vi "Tree.vi"   [LabVIEW 2011, in "Messenging.lvlib"]
doc: "Commonly used VI's."
uses:
  Messenging.lvlib
  Interprocess Messenger/QueueMessenger/QueueMessenger.lvclass
  Interprocess Messenger/EventMessenger/EventMessenger.lvclass
  Interprocess Messenger/Messenger (Parent)/MGR.lvclass
  Interprocess Messenger/Send/Send.lvclass
  Interprocess Messenger/Send/Send Message.vi
  Interprocess Messenger/TextVarientMessage/MSG.lvclass
  Parallel Process/Parallel Process.lvclass
  Parallel Process/Messsage Logger/Message Logger.lvclass
  Parallel Process/State Logger Folder/State Logger.lvclass
  Parallel Process/PP Template (Receive type)/PP Template.lvclass
  Parallel Process/PP Template (EventUI)/Parallel Process Template (EventUI) Folder/PP Template (UserEvent).lvclass
  Interprocess Messenger/SendMultiple/Create Observer.vi
  Interprocess Messenger/SendMultiple/ObserverSet.lvclass
  Interprocess Messenger/SendOnly/Observer.lvclass
  Parallel Process/ObserverRegister/ObserverRegistry.lvclass
  Parallel Process/ObserverRegister/Menu/Notify Observers (State).vi
  Interprocess Messenger/Cancelable Observer/CancelableObserver.lvclass
  Parallel Process/Metronome/Metronome.lvclass
  Interprocess Messenger/TextVarientMessage/Reply (message).vi
  Interprocess Messenger/TextVarientMessage/Write (no data).vi
  Interprocess Messenger/Send/Query (static).vi
  Parallel Process/Attach Observer.vi
  Interprocess Messenger/Receiver/MGR (Receive type).lvclass
  Interprocess Messenger/VarMessage/Extract Varient (static).vi
panel:
  # "See diagram"
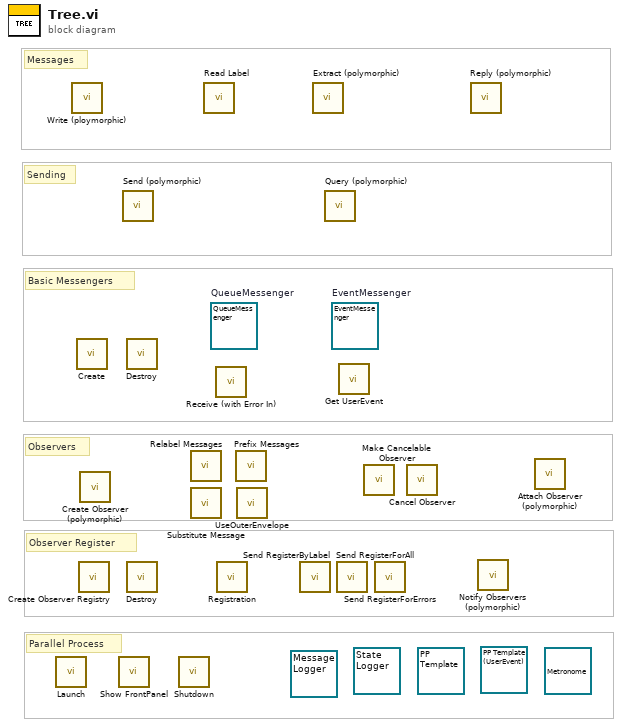
[diagram p0: block diagram]
diagram:
  (unwired) refnum<class "Metronome.lvclass"> refnum ("Messenging.lvlib:Metronome.lvclass")
  (unwired) refnum<class "PP Template (UserEvent).lvclass"> refnum ("Messenging.lvlib:PP Template (UserEvent).lvclass")
  (unwired) refnum<class "PP Template.lvclass"> refnum ("Messenging.lvlib:PP Template.lvclass")
  (unwired) refnum<class "State Logger.lvclass"> refnum ("Messenging.lvlib:State Logger.lvclass")
  (unwired) refnum<class "Message Logger.lvclass"> refnum ("Messenging.lvlib:Message Logger.lvclass")
  (unwired) refnum<class "EventMessenger.lvclass"> refnum  # EventMessenger
  (unwired) refnum<class "QueueMessenger.lvclass"> refnum  # QueueMessenger
  # "Parallel Process"
  # "Observer Register"
  # "Observers"
  # "Basic Messengers"
  # "Sending"
  # "Messages"
  n1 = call-dynamic "Launch.vi"() -> ()  [unwired: 9 in, 3 out]
  n2 = call-poly "Write (ploymorphic).vi"() -> ()  [unwired: 10 in, 2 out]
  n3 = call-dynamic "Create.vi"() -> ()  [unwired: 10 in, 2 out]
  n4 = call "Create Observer Registry.vi"() -> ()  [unwired: 10 in, 2 out]
  n5 = call-poly "Create Observer (polymorphic).vi"() -> ()  [unwired: 9 in, 1 out]
  n6 = call-dynamic "Show FrontPanel.vi"() -> ()  [unwired: 10 in, 2 out]
  n7 = call-poly "Send (polymorphic).vi"() -> ()  [unwired: 10 in, 2 out]
  n8 = call-dynamic "Destroy.vi"() -> ()  [unwired: 11 in, 1 out]
  n9 = call "Destroy.vi"() -> ()  [unwired: 10 in, 2 out]
  n10 = call-dynamic "Shutdown.vi"() -> ()  [unwired: 10 in, 2 out]
  n11 = call "Relabel Messages.vi"() -> ()  [unwired: 11 in, 1 out]
  n12 = call "Substitute Message.vi"() -> ()  [unwired: 11 in, 1 out]
  n13 = call-dynamic "Read Label.vi"() -> ()  [unwired: 9 in, 3 out]
  n14 = call-dynamic "Receive (with Error In).vi"() -> ()  [unwired: 8 in, 4 out]
  n15 = call "Registration.vi"() -> ()  [unwired: 9 in, 3 out]
  n16 = call "Prefix Messages.vi"() -> ()  [unwired: 11 in, 1 out]
  n17 = call "UseOuterEnvelope.vi"() -> ()  [unwired: 11 in, 1 out]
  n18 = call "Send RegisterByLabel.vi"() -> ()  [unwired: 10 in, 2 out]
  n19 = call-poly "Extract (polymorphic).vi"() -> ()  [unwired: 8 in, 4 out]
  n20 = call-poly "Query (polymorphic).vi"() -> ()  [unwired: 9 in, 3 out]
  n21 = call "Send RegisterForAll.vi"() -> ()  [unwired: 10 in, 2 out]
  n22 = call-dynamic "Get UserEvent.vi"() -> ()  [unwired: 9 in, 3 out]
  n23 = call "Make Cancelable Observer.vi"() -> ()  [unwired: 10 in, 2 out]
  n24 = call "Send RegisterForErrors.vi"() -> ()  [unwired: 10 in, 2 out]
  n25 = call "Cancel Observer.vi"() -> ()  [unwired: 11 in, 1 out]
  n26 = call-poly "Reply (polymorphic).vi"() -> ()  [unwired: 10 in, 2 out]
  n27 = call-poly "Notify Observers (polymorphic).vi"() -> ()  [unwired: 10 in, 2 out]
  n28 = call-poly "Attach Observer (polymorphic).vi"() -> ()  [unwired: 11 in, 1 out]
